vi "Przenies mnozniki konw FVG.vi"(7 "Akcja (GET)":T4, 8 "error in (no error)":errorcluster, 10 "No":i32, 11 "Przetwornik in":T1={"Numer"=1, "Opis"="Kanał 1", "Zakres"=enum."1000V", "Filtr"=FALSE, "Typ pomiaru"=enum."Pomiar DC", "Aktywny"=FALSE, "Wartość"={"X"="U", "[ ]"="V", "trans X"=1.0, "trans U"=1.0, "Z tabeli"=FALSE, "Opis"=""}} {"Numer" min=1 max=8 step=1}) -> (0 "error out":errorcluster, 2 "Konw mnozniki":dbl[](array[numeric]))   [LabVIEW 2014]
doc: "Oblicza wartościmnożników wynikających z zastosowanego konwertera"
uses:
  Kontrolki/FVGs/FVG akwizycje akcje.ctl
  Kontrolki/GUI/AI_parametry.ctl
  Kontrolki/GUI/AI_typ pom.ctl
  Kontrolki/GUI/AI_wartosc.ctl
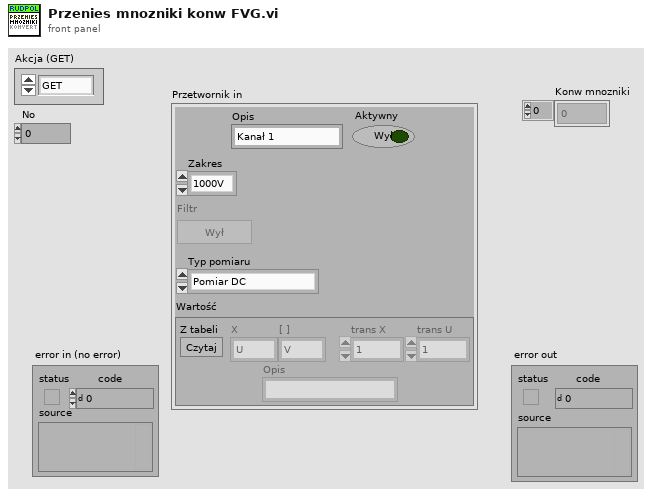
[diagram p1: front panel]
types:
  T1 = typedef "AI_parametry.ctl" = cluster{"Numer":u8, "Opis":string, "Zakres":enum16{"1000V", "300V", "30V", "3V", "0,3V"}, "Filtr":bool, "Typ pomiaru":T2, "Aktywny":bool, "Wartość":T3}
  T2 = typedef "AI_typ pom.ctl" = enum16{"Pomiar DC", "Pomiar AC+DC", "Pomiar AC"}
  T3 = typedef "AI_wartosc.ctl" = cluster{"X":string, "[ ]":string, "trans X":dbl, "trans U":dbl, "Z tabeli":bool, "Opis":string}
  T4 = typedef "FVG akwizycje akcje.ctl" = enum16{"GET", "GETr", "SET"}
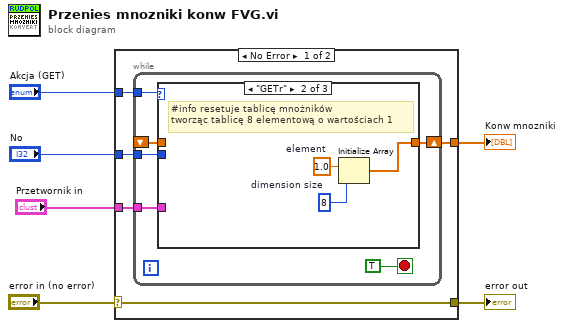
[diagram p0: block diagram]
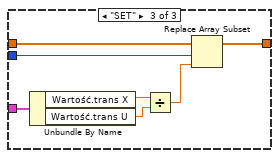
[diagram p3: hidden frame]
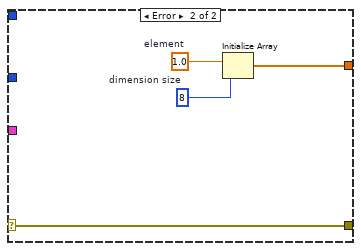
[diagram p4: hidden frame]
diagram:
  n1 = case shown="No Error" "error in (no error)" {
    selector: "error in (no error)" -> [w7 w32]
    tunnel: [w7 w32] -> w5
    tunnel: "Przetwornik in" -> [w9 _]
    tunnel: "Akcja (GET)" -> [w11 _]
    tunnel: "No" -> [w10 _]
    tunnel: [w8 w29] -> w2
    frame No Error {
      n2 = while {
        tunnel: w11 -> [w16]
        shift-right: [w15] -> w8
        shift-left: _ -> [w14]
        tunnel: w10 -> [w13]
        tunnel: w9 -> [w12]
        stop <- TRUE stop-if-true
        n3 = case shown="\"GETr\"" w16 {
          tunnel: [w18 w19 w27] -> w15
          tunnel: w14 -> [w18 _ w28]
          tunnel: w13 -> [_ _ w26]
          tunnel: w12 -> [_ _ w25]
          frame "GET", Default {
          }
          frame "GETr" {
            w20 = 8  # dimension size
            w21 = 1.0  # element
            # "#info resetuje tablicę mnożników\ntworząc tablicę 8 elementową o wartościach 1"
            n4 = Initialize Array(w21, w20) -> (w19:dbl[])
          }
          frame "SET" {
            n5 = Unbundle By Name(w25) -> ("Wartość.trans X"=w24:dbl, "Wartość.trans U"=w23:dbl)
            n6 = Divide(x=w24, y=w23) -> (x/y=w22:dbl)
            n7 = Replace Array Subset(array=w28, new element=w22, index=w26) -> (w27:dbl[])
          }
        }
      }
    }
    frame Error {
      w31 = 8  # dimension size
      w30 = 1.0  # element
      n8 = Initialize Array(w30, w31) -> (w29:dbl[])
    }
  }
  "error out" <- w5
  "Konw mnozniki" <- w2
